vi "CAEN_CUR_SET (SubVI).vi"(7 "Numeric":dbl, 8 "error in (no error)":errorcluster, 10 "CHANNEL":string(combo), 11 "Cluster in 2":T1={"BAUDE RATE"=enum."9600", "VISA RESOURCE NAME"=""}) -> (0 "error out":errorcluster)   [LabVIEW 2020]
uses:
  Desktop/eTPC/subVIs for MKS/INITIALIZATION PFEIFFER.ctl
  <vilib>/Instr/_visa.llb/VISA Configure Serial Port (Instr).vi
panel:
  out "result string":string
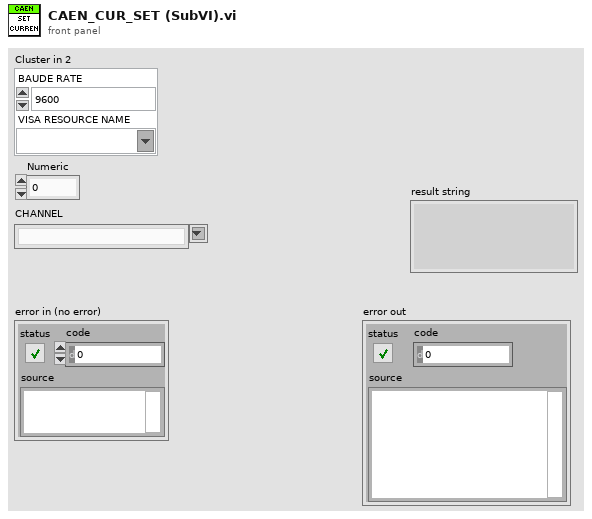
[diagram p1: front panel]
types:
  T1 = typedef "INITIALIZATION PFEIFFER.ctl" = cluster{"BAUDE RATE":enum32{"38400", "19200", "9600", "4800"}, "VISA RESOURCE NAME":refnum<visa-resource-name>}
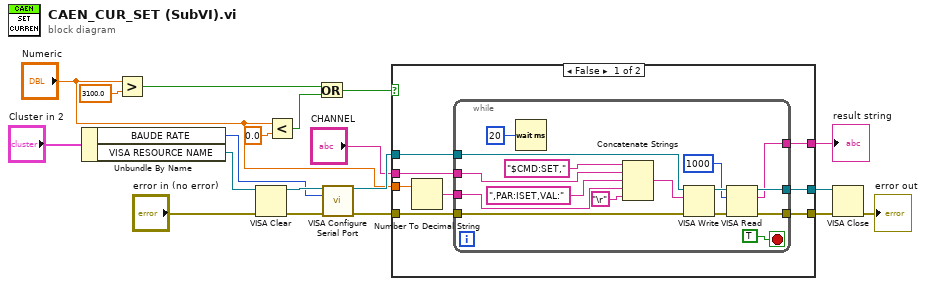
[diagram p0: block diagram]
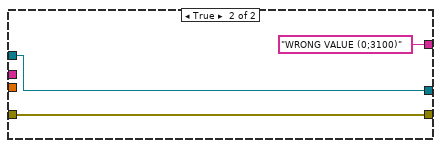
[diagram p2: hidden frame]
diagram:
  n1 = Unbundle By Name("Cluster in 2") -> ("BAUDE RATE"=w1:enum32{"38400", "19200", "9600", "4800"}, "VISA RESOURCE NAME"=w2:refnum<visa-resource-name>)
  n2 = Greater?(x="Numeric", y=3100.0) -> (0:w11:bool)
  n3 = VISA Clear(VISA resource name=w2, error in (no error)="error in (no error)") -> (VISA resource name out=w6:refnum<visa-resource-name>, error out=w5:errorcluster)
  n4 = Less?(x="Numeric", y=0.0) -> (x < y?=w10:bool)
  n5 = Or(x=w11, y=w10) -> (x .or. y?=w9:bool)
  n6 = call-poly "VISA Configure Serial Port"("VISA resource name"=w6, "baud rate (9600)"=w1, "error in (no error)"=w5) -> ("VISA resource name out"=w19:refnum<visa-resource-name>, "error out"=w18:errorcluster)  [unwired: 11 in]
  n7 = case shown="False" w9 {
    tunnel: w19 -> [w27 w46]
    tunnel: w18 -> [w26 w45]
    tunnel: [w25 w46] -> w17
    tunnel: [w24 w45] -> w16
    tunnel: "CHANNEL" -> [w23 _]
    tunnel: "Numeric" -> [w21 _]
    tunnel: [w20 "WRONG VALUE (0;3100)" ("result string")] -> w7
    frame False {
      n8 = Number To Decimal String(number=w21) -> (decimal integer string=w22:string)  [unwired: 1 in]
      n9 = while {
        tunnel: w27 -> [w43]
        tunnel: w26 -> [w42]
        tunnel: [w37] -> w24
        tunnel: [w36] -> w25
        tunnel: w23 -> [w31]
        tunnel: w22 -> [w29]
        tunnel: [w28] -> w20
        stop <- TRUE stop-if-true
        n10 = Wait (ms)(milliseconds to wait=u32 20) -> ()  [unwired: 1 out]
        n11 = Concatenate Strings("$CMD:SET," ("string"), w31, ",PAR:ISET,VAL:" ("string"), w29, "\r") -> (w34:string)
        n12 = VISA Write(VISA resource name=w43, write buffer=w34, error in (no error)=w42) -> (VISA resource name out=w39:refnum<visa-resource-name>, error out=w38:errorcluster)  [unwired: 1 out]
        n13 = VISA Read(VISA resource name=w39, byte count=u32 1000, error in (no error)=w38) -> (VISA resource name out=w36:refnum<visa-resource-name>, read buffer=w28:string, error out=w37:errorcluster)  [unwired: 1 out]
      }
    }
    frame True {
    }
  }
  "result string" <- w7
  n14 = VISA Close(VISA resource name=w17, error in (no error)=w16) -> (error out=→"error out":errorcluster)
